vi "Load Function.vi"(8 "error in (no error)":errorcluster, 11 "Instrument in":refnum<class "Instrument.lvclass">) -> (0 "error out":errorcluster, 3 "Instrument out":refnum<class "Instrument.lvclass">)   [LabVIEW 2018, in "Instrument.lvclass"]
uses:
  Instrument.lvclass
  Instrument.lvclass/Instrument.ctl
  Device/Optics/Optics.lvclass/Optics.ctl
  Device/Optics/Opt_Selector/Opt_Selector.lvclass
  C:/Users/devstaff/sparc4/s4gui/Versao ZeroMQ REQ-REP/SPARC4_GUI -v1.0.0 - 20250122_ICS-JSON/Device/Optics/Optics.lvclass
  Device/Optics/Optics.lvclass
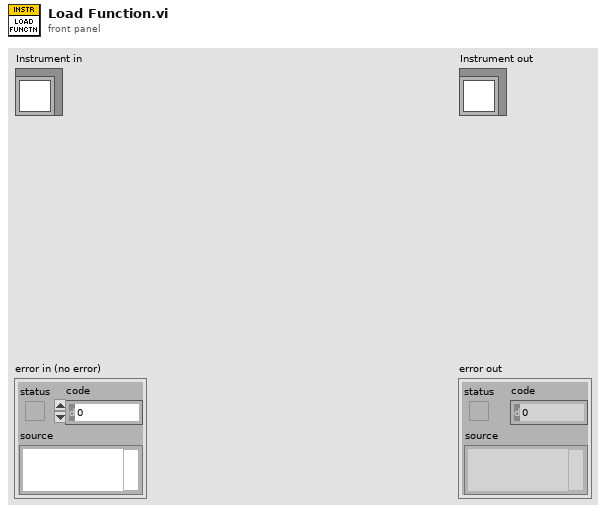
[diagram p1: front panel]
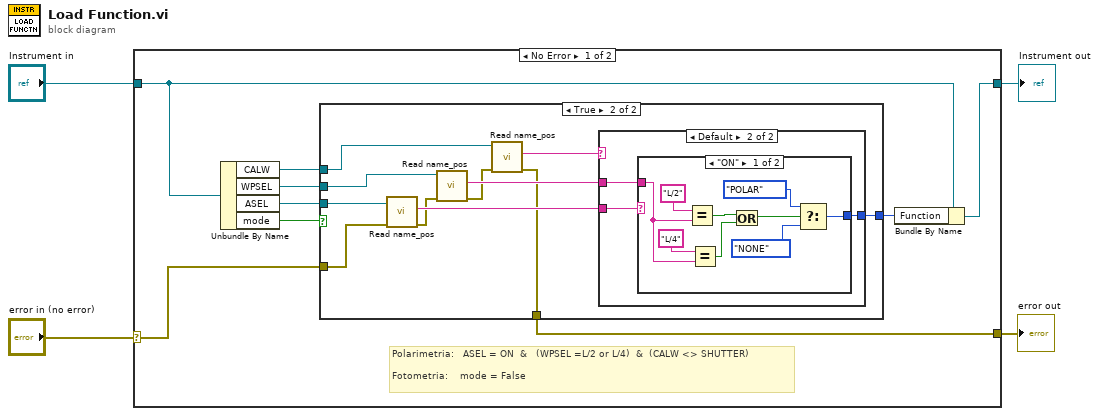
[diagram p0: block diagram]
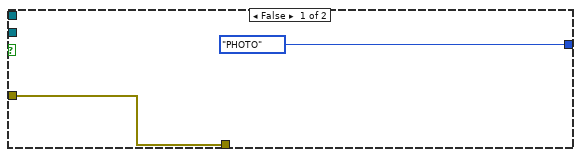
[diagram p2: hidden frame]
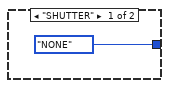
[diagram p3: hidden frame]
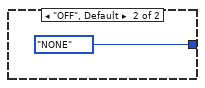
[diagram p4: hidden frame]
diagram:
  n1 = case shown="No Error" "error in (no error)" {
    selector: "error in (no error)" -> [w8 w42]
    tunnel: [w6 w42] -> w3
    tunnel: [w12 w41] -> w1
    tunnel: "Instrument in" -> [w13 w41]
    frame No Error {
      # "Polarimetria:   ASEL = ON  &   (WPSEL =L/2 or L/4)  &  (CALW <> SHUTTER) \n\nFotometria:    mode = False"
      n2 = Unbundle By Name(w13) -> ("CALW"=w5:refnum<class "Opt_Selector.lvclass">, "WPSEL"=w7:refnum<class "Opt_Selector.lvclass">, "ASEL"=w9:refnum<class "Opt_Selector.lvclass">, "mode"=w10:bool)
      n3 = case shown="True" w10 {
        tunnel: [enum16{"PHOTO", "POLAR", "NONE"}."PHOTO" ("Function") w23] -> w11
        tunnel: w9 -> [_ w26]
        tunnel: w8 -> [w14 w25]
        tunnel: w7 -> [_ w21]
        tunnel: [w14 w17] -> w6
        tunnel: w5 -> [_ w19]
        frame False {
        }
        frame True {
          n4 = call "Read name_pos.vi"("error in (no error)"=w25, "Optics in"=w26) -> ("error out"=w22:errorcluster, "name_pos"=w24:string)  [unwired: 7 in, 1 out]
          n5 = call "Read name_pos.vi"("error in (no error)"=w22, "Optics in"=w21) -> ("error out"=w18:errorcluster, "name_pos"=w20:string)  [unwired: 7 in, 1 out]
          n6 = call "Read name_pos.vi"("error in (no error)"=w18, "Optics in"=w19) -> ("error out"=w17:errorcluster, "name_pos"=w16:string)  [unwired: 7 in, 1 out]
          n7 = case shown="Default" w16 {
            tunnel: w24 -> [_ w30]
            tunnel: [enum16{"PHOTO", "POLAR", "NONE"}."NONE" ("Function") w29] -> w23
            tunnel: w20 -> [_ w28]
            frame "SHUTTER" {
            }
            frame Default {
              n8 = case shown="\"ON\"" w30 {
                tunnel: [w34 enum16{"PHOTO", "POLAR", "NONE"}."NONE" ("Function")] -> w29
                tunnel: w28 -> [w35 _]
                frame "ON" {
                  n9 = Equal?(x="L/2" ("Boolean Text.Text"), y=w35) -> (x = y?=w38:bool)
                  n10 = Equal?(x="L/4" ("Boolean Text.Text"), y=w35) -> (x = y?=w36:bool)
                  n11 = Or(x=w38, y=w36) -> (x .or. y?=w32:bool)
                  n12 = Select(t=enum16{"PHOTO", "POLAR", "NONE"}."POLAR" ("Function"), s=w32, f=enum16{"PHOTO", "POLAR", "NONE"}."NONE" ("Function")) -> (s? t:f=w34:enum16{"PHOTO", "POLAR", "NONE"})
                }
                frame "OFF", Default {
                }
              }
            }
          }
        }
      }
      n13 = Bundle By Name(cluster=w13, "Function"=w11) -> (w12:refnum<class "Instrument.lvclass">)
    }
    frame Error {
    }
  }
  "error out" <- w3
  "Instrument out" <- w1
